vi "FL Get Membership Function Names.vi"   [LabVIEW 2017, in "NI_Fuzzy_Logic_API.lvlib"]
doc: "Returns the names of the linguistic terms for a linguistic variable. Membership functions represent the degree of membership of linguistic variables within their linguistic terms. You can return the names of the membership functions from a fuzzy system or from an array of membership functions. The data type you wire to the <B>fuzzy system in</B> input determines the polymorphic instance to use."
uses:
  <vilib>/addons/Fuzzy Logic/NI_Fuzzy_Logic_API.lvlib
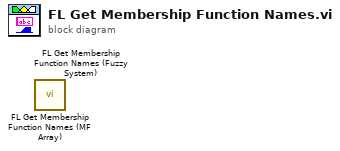
[diagram p0: block diagram]
diagram:
  n1 = call <vilib>:"FL Get Membership Function Names (MF Array).vi"() -> ()  [unwired: 9 in, 3 out]
  n2 = call <vilib>:"FL Get Membership Function Names (Fuzzy System).vi"() -> ()  [unwired: 9 in, 3 out]
